vi "Global 2.vi"() -> ()   [LabVIEW 2011]
panel:
  out "Effective field 2":dbl[unit] format="%.3f"
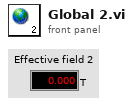
[diagram p1: front panel]
diagram:
